vi "Spartan HTTP Log Error.vi"(4 "error in (no error)":errorcluster, 6 "authorization addr":string, 7 "message":string) -> (0 "error out":errorcluster)   [LabVIEW 2011]
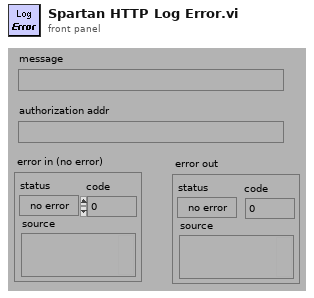
[diagram p1: front panel]
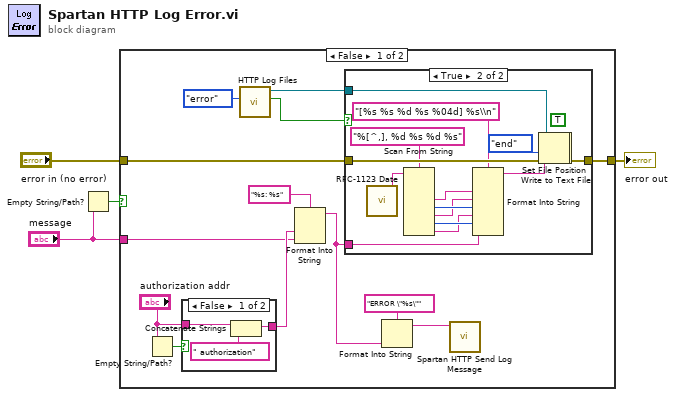
[diagram p0: block diagram]
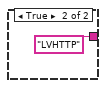
[diagram p3: hidden frame]
diagram:
  n1 = Empty String/Path?(string/path="message") -> (empty?=w1:bool)
  n2 = case shown="False" w1 {
    tunnel: "message" -> [w10 _]
    tunnel: "error in (no error)" -> [w9 w39]
    tunnel: [w15 w39] -> w2
    frame False {
      n3 = Empty String/Path?(string/path="authorization addr") -> (empty?=w17:bool)
      n4 = case shown="False" w17 {
        tunnel: "authorization addr" -> [w37 _]
        tunnel: [w35 "LVHTTP"] -> w11
        frame False {
          n5 = Concatenate Strings(w37, " authorization") -> (w35:string)
        }
        frame True {
        }
      }
      n6 = call "HTTP Log Files.vi"("log file (error)"=enum16{"error", "transfer", "agent", "referer"}."error") -> ("valid refnum"=w12:bool, "refnum"=w13:refnum<file>)  [unwired: 2 in, 3 out]
      n7 = Format Into String(format string="%s: %s", w11, w10) -> (resulting string=w6:string)  [unwired: 2 in, 1 out]
      n8 = case shown="True" w12 {
        tunnel: w13 -> [_ w34]
        tunnel: [w18 w32] -> w15
        tunnel: w9 -> [w18 w31]
        tunnel: w6 -> [_ w21]
        frame False {
        }
        frame True {
          (unwired) TRUE ("convert eol (F)")
          n9 = call "RFC-1123 Date.vi"() -> ("GMT Date/Time"=w30:string)  [unwired: 1 in, 1 out]
          n10 = Scan From String(format string="%[^,], %d %s %d %s", input string=w30) -> (output 1=w25:string, output 2=w27:i32, output 3=w26:string, output 4=w29:i32, output 5=w28:string)  [unwired: 2 in, 8 out]
          n11 = Format Into String(format string="[%s %s %d %s %04d] %s\\n", w25, w26, w27, w28, w29, w21) -> (resulting string=w22:string)  [unwired: 2 in, 1 out]
          n12 = Set File Position(refnum=w34, from (0:start)=enum16{"start", "end", "current"}."end" ("pos mode (0:2)"), error in=w31) -> (refnum out=w20:refnum<file>, error out=w19:errorcluster)  [unwired: 1 out]
          n13 = Write to Text File(file (use dialog)=w20, text=w22, error in=w19) -> (error out=w32:errorcluster)  [unwired: 3 out]
        }
      }
      n14 = Format Into String(format string="ERROR \"%s\"", w6) -> (resulting string=w5:string)  [unwired: 2 in, 1 out]
      n15 = call "Spartan HTTP Send Log Message.vi"("message"=w5) -> ()  [unwired: 7 out]
    }
    frame True {
    }
  }
  "error out" <- w2
